vi "close.vi"(8 "error in":errorcluster, 11 "Modbus Slave runtime in":refnum<class "Modbus Slave runtime.lvclass">) -> (0 "error out":errorcluster)   [LabVIEW 2013, in "Modbus Slave runtime.lvclass"]
doc: "Provides an interface for terminating a module instance. While this interface performs no operations, a child should close and deallocate any open references or memory.Platypus Framework 1.0.1.65\nNI Systems Engineering - National Instruments"
uses:
  Modbus Slave runtime.lvclass
  Modbus Slave runtime.lvclass/Modbus Slave runtime.ctl
  <vilib>/NI/Modbus Library/API/Slave/Modbus Slave.lvclass
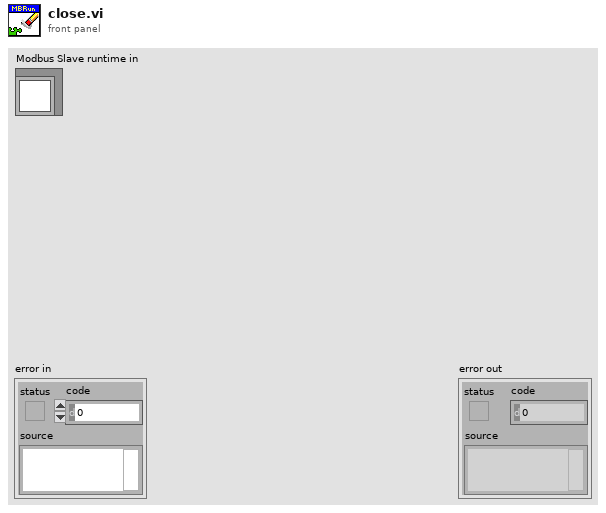
[diagram p1: front panel]
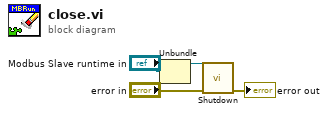
[diagram p0: block diagram]
diagram:
  n1 = Unbundle("Modbus Slave runtime in") -> (w1:refnum<class "Modbus Slave.lvclass">)  [unwired: 2 out]
  n2 = call-dynamic "Shutdown.vi"("error in"="error in", "Modbus slave in"=w1) -> ("error out"=→"error out":errorcluster)  [unwired: 9 in]
